vi "speakerCenterData.vi"() -> (7 "DistanceToTarget (Inch)":dbl, 8 "Target Yaw":dbl, 9 "Yaw Offset (Degrees)":dbl, 10 "Target?":bool)   [LabVIEW 2023]
uses:
  <vilib>/Rock Robotics/WPI/ThirdParty/PhotonVisionLib/SubVI/PhotonPipelineResult_Unpack.vi
  <vilib>/Rock Robotics/WPI/ThirdParty/PhotonVisionLib/SubVI/PhotonPipelineResult_SetTimeStampSecs.vi
  <vilib>/Rock Robotics/WPI/ThirdParty/PhotonVisionLib/SubVI/PhotonPipelineResult_GetLatency_Millis.vi
  <vilib>/Rock Robotics/WPI/ThirdParty/JAS_Junk/TrajLib/Util_GetTime.vi
  <vilib>/Rock Robotics/WPI/ThirdParty/PhotonVisionLib/SubVI/PhotonPipelineResult_GetTimeStampSecs.vi
  <vilib>/Rock Robotics/WPI/ThirdParty/PhotonVisionLib/SubVI/Packet_decode_Flt64.vi
  <vilib>/Rock Robotics/WPI/ThirdParty/PhotonVisionLib/SubVI/Packet_decode_ByteI8.vi
  <vilib>/Rock Robotics/WPI/ThirdParty/PhotonVisionLib/SubVI/PhotonTrackedTarget_Unpack.vi
  <vilib>/Rock Robotics/WPI/ThirdParty/PhotonVisionLib/SubVI/PhotonMultiTargetPNPResult_unpack.vi
  <vilib>/Rock Robotics/WPI/ThirdParty/PhotonVisionLib/SubVI/PhotonPipelineResult_New.vi
  <vilib>/Rock Robotics/WPI/ThirdParty/JAS_Junk/TrajLib/VI/Util_GetTime_U32.vi
  <vilib>/Rock Robotics/WPI/ThirdParty/PhotonVisionLib/SubVI/TargetCorner_New.vi
  <vilib>/Rock Robotics/WPI/ThirdParty/PhotonVisionLib/SubVI/Packet_decode_Int32.vi
  <vilib>/Rock Robotics/WPI/ThirdParty/PhotonVisionLib/SubVI/Packet_decode_Transform3d.vi
  <vilib>/Rock Robotics/WPI/ThirdParty/PhotonVisionLib/SubVI/PhotonPNPResult_unpackt.vi
  <vilib>/Rock Robotics/WPI/ThirdParty/PhotonVisionLib/SubVI/PhotonMultiTargetPNPResult_New.vi
  <vilib>/Rock Robotics/WPI/ThirdParty/PhotonVisionLib/SubVI/PhotonMultiTargetPNPResult_MAX_IDS.vi
  <vilib>/Rock Robotics/WPI/ThirdParty/PhotonVisionLib/SubVI/Packet_decode_Int16.vi
  <vilib>/Rock Robotics/WPI/ThirdParty/JAS_Junk/TrajLib/VI/Transform3d_Create_Trans3dRot3d.vi
  <vilib>/Rock Robotics/WPI/ThirdParty/JAS_Junk/TrajLib/VI/Translation3d_Create.vi
  <vilib>/Rock Robotics/WPI/ThirdParty/JAS_Junk/TrajLib/VI/Rotation3d_Create_Quaternion.vi
  <vilib>/Rock Robotics/WPI/ThirdParty/JAS_Junk/TrajLib/VI/Quaternion_New.vi
  <vilib>/Rock Robotics/WPI/ThirdParty/PhotonVisionLib/SubVI/Packet_decode_Boolean.vi
  <vilib>/Rock Robotics/WPI/ThirdParty/PhotonVisionLib/SubVI/PhotonPNPResult_New_Empty.vi
  <vilib>/Rock Robotics/WPI/ThirdParty/PhotonVisionLib/SubVI/PhotonPNPResult_New.vi
  <vilib>/Rock Robotics/WPI/ThirdParty/JAS_Junk/TrajLib/VI/Quaternion_Normalize.vi
  <vilib>/Rock Robotics/WPI/ThirdParty/JAS_Junk/TrajLib/VI/Quaternion_New_Default.vi
  <vilib>/Rock Robotics/Network Tables/NT Read Value.vi
  <vilib>/Rock Robotics/Network Tables/NT Read Raw.vi
  <vilib>/Rock Robotics/SystemInterfaces/Utilities/FPGA_UtilitiesRead LocalTime.vi
  <vilib>/Rock Robotics/WPI/ThirdParty/JAS_Junk/TrajLib/VI/Util_GetTime_U64.vi
  <vilib>/Rock Robotics/WPI/ThirdParty/PhotonVisionLib/PhotonVisionLib.lvlib
  <vilib>/Rock Robotics/WPI/ThirdParty/JAS_Junk/TrajLib/Trajectory_Library.lvlib
panel:
  in  "Gyro Reading (Deg)":dbl
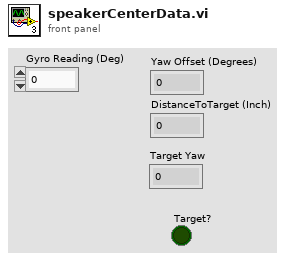
[diagram p1: front panel]
types:
  T1 = typedef "PhotonVisionLib.lvlib/PhotonPipelineResultType.ctl" = cluster{"TargetCount":i32, "Latency_MilliSec":dbl, "Targets":T2[], "TimeStampSec":dbl, "PhotonMultiTargetPNPResult":T8}
  T2 = typedef "PhotonVisionLib.lvlib/PhotonTrackedTargetType.ctl" = cluster{"Yaw":dbl, "Pitch":dbl, "Area":dbl, "Skew":dbl, "MinAreaRectCorners":T3[], "BestCameraToTarget":T4, "FiiducialId":i32, "AltCameraToTarget":T4, "PoseAmbiguity":dbl, "DetectedCorners":T3[]}
  T3 = typedef "PhotonVisionLib.lvlib/TargetCornerType.ctl" = cluster{"X":dbl, "Y":dbl}
  T4 = typedef "Trajectory_Library.lvlib/TRANSFORM3D.ctl" = cluster{"TRANSLATION3D":T5, "ROTATION3D":T6, "XF":bool}
  T5 = typedef "Trajectory_Library.lvlib/TRANSLATION3D.ctl" = cluster{"X":dbl, "Y":dbl, "Z":dbl}
  T6 = typedef "Trajectory_Library.lvlib/ROTATION3D.ctl" = cluster{"Q_quaternion":T7}
  T7 = typedef "Trajectory_Library.lvlib/QUATERNION.ctl" = cluster{"R":dbl, "V":dbl[]}
  T8 = typedef "PhotonVisionLib.lvlib/PhotonMultiTargetPNPResultType.ctl" = cluster{"PhotonPNPResult":T9, "FiducialIDsUsed":i16[]}
  T9 = typedef "PhotonVisionLib.lvlib/PhotonPNPResultType.ctl" = cluster{"IsPresent":bool, "bestReprojErr":dbl, "altReprojErr":dbl, "ambiguity":dbl, "Best":T4, "Alt":T4}
  T10 = typedef "WPI_DriverStationAllianceInfo.ctl" = enum16{"Red", "Blue", "Invalid"}
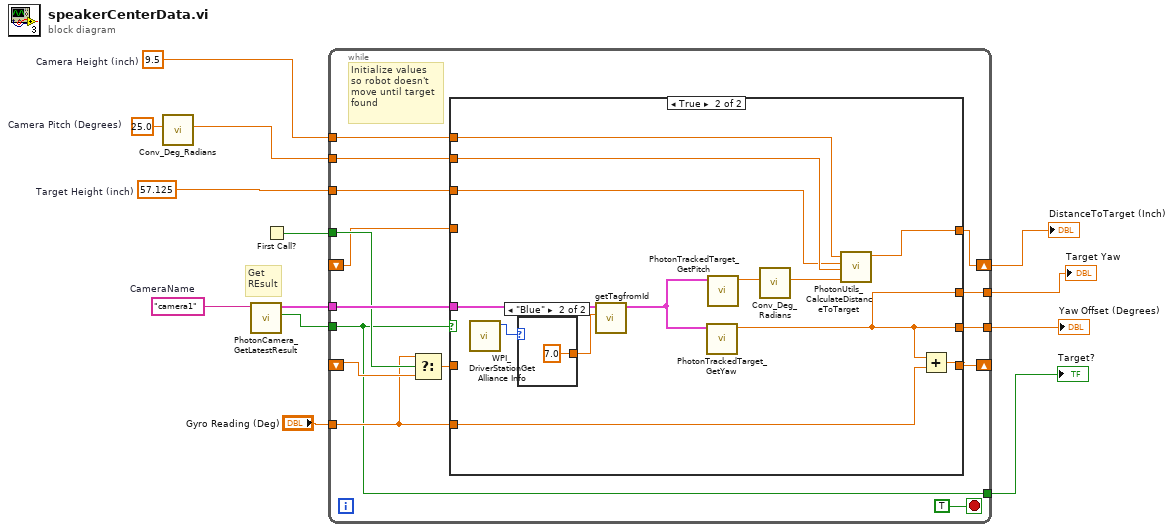
[diagram p0: block diagram]
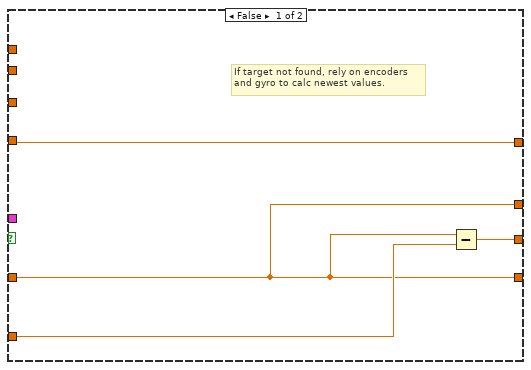
[diagram p2: hidden frame]
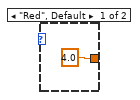
[diagram p3: hidden frame]
diagram:
  w10 = 57.125  # Target Height (inch)
  w8 = 9.5  # Camera Height (inch)
  w5 = 25.0  # Camera Pitch (Degrees)
  w4 = "camera1"  # CameraName
  # "Get\nREsult"
  n1 = call <vilib>:"Conv_Deg_Radians.vi"("Degress"=w5) -> ("Radians"=w9:dbl)  [unwired: 10 in]
  n2 = call <vilib>:"PhotonCamera_GetLatestResult.vi"("CameraName"=w4) -> ("HasTargets"=w6:bool, "PipelineResult"=w7:T1)  [unwired: 7 in, 2 out]
  n3 = First Call?() -> (First Call?: T/F=w13:bool)
  n4 = while {
    tunnel: w6 -> [w14]
    tunnel: w7 -> [w28]
    tunnel: w8 -> [w27]
    tunnel: w9 -> [w26]
    tunnel: w10 -> [w25]
    tunnel: [w23] -> w1
    tunnel: "Gyro Reading (Deg)" -> [w17]
    shift-right: [w21] -> _
    shift-left: _ -> [w20]
    tunnel: w13 -> [w18]
    shift-right: [w24] -> w11
    shift-left: _ -> [w16]
    tunnel: [w15] -> w3
    tunnel: [w14] -> w2
    stop <- TRUE stop-if-true
    # "Initialize values\nso robot doesn't\nmove until target\nfound"
    n5 = Select(t=w17, s=w18, f=w20) -> (s? t:f=w19:dbl)
    n6 = case shown="True" w14 {
      tunnel: w28 -> [_ w37]
      tunnel: [w32 w33] -> w23
      tunnel: w27 -> [_ w43]
      tunnel: w26 -> [_ w42]
      tunnel: w25 -> [_ w41]
      tunnel: [w30 w40] -> w24
      tunnel: w17 -> [w31 w39]
      tunnel: [w29 w38] -> w21
      tunnel: w19 -> [w29 _]
      tunnel: w16 -> [w30 _]
      tunnel: [w29 w33] -> w15
      frame False {
        # "If target not found, rely on encoders\nand gyro to calc newest values."
        n7 = Subtract(x=w29, y=w31) -> (x-y=w32:dbl)
      }
      frame True {
        n8 = call <vilib>:"WPI_DriverStationGet Alliance Info.vi"() -> ("Alliance"=w36:T10)  [unwired: 6 in, 5 out]
        n9 = case shown="\"Blue\"" w36 {
          tunnel: [4.0 ("Numeric") 7.0 ("Numeric")] -> w35
          frame "Red", Default {
          }
          frame "Blue" {
          }
        }
        n10 = call "getTagfromId.vi"("ID"=w35, "PipelineResult"=w37) -> ("PhotonTrackedTarget"=w34:T2)  [unwired: 9 in]
        n11 = call <vilib>:"PhotonTrackedTarget_GetYaw.vi"("TrackedTarget"=w34) -> ("Yaw"=w33:dbl)  [unwired: 10 in]
        n12 = call <vilib>:"PhotonTrackedTarget_GetPitch.vi"("TrackedTarget"=w34) -> ("Pitch"=w45:dbl)  [unwired: 10 in]
        n13 = call <vilib>:"Conv_Deg_Radians.vi"("Degress"=w45) -> ("Radians"=w44:dbl)  [unwired: 10 in]
        n14 = call <vilib>:"PhotonUtils_CalculateDistanceToTarget.vi"("TargetPitch_Radians"=w44, "CameraPitch_Radians"=w42, "TargetHeight_Inch"=w41, "CameraHeight_Inch"=w43) -> ("DistanceToTarget_Inch"=w40:dbl)  [unwired: 7 in]
        n15 = Add(x=w33, y=w39) -> (x+y=w38:dbl)
      }
    }
  }
  "DistanceToTarget (Inch)" <- w11
  "Yaw Offset (Degrees)" <- w1
  "Target Yaw" <- w3
  "Target?" <- w2
